vi "Que.-startvalue for Serial Input.vi"() -> (0 "error out":errorcluster, 1 "queue out":refnum<queue>)   [LabVIEW 2016]
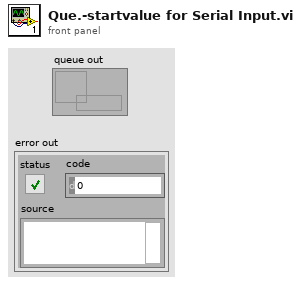
[diagram p1: front panel]
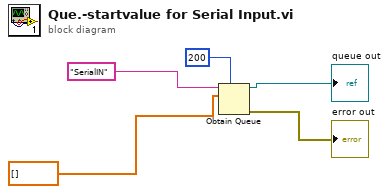
[diagram p0: block diagram]
diagram:
  n1 = Obtain Queue(max queue size (-1, unlimited)=200, name (unnamed)="SerialIN", element data type=dbl[] []) -> (queue out=→"queue out":refnum<queue>, error out=→"error out":errorcluster)  [unwired: 2 in, 1 out]
